vi "Rasnik_Discrepancy.vi"(7 "angle array":string[](array[string]), 8 "pattern":string, 9 "path":path, 10 "Y array":string[](array[string]), 11 "X array":string[](array[string])) -> (1 "angle discrepancy":dbl[](array[numeric]), 2 "Y discrepancy":dbl[](array[numeric]), 3 "X discrepancy":dbl[](array[numeric]))   [LabVIEW 2015]
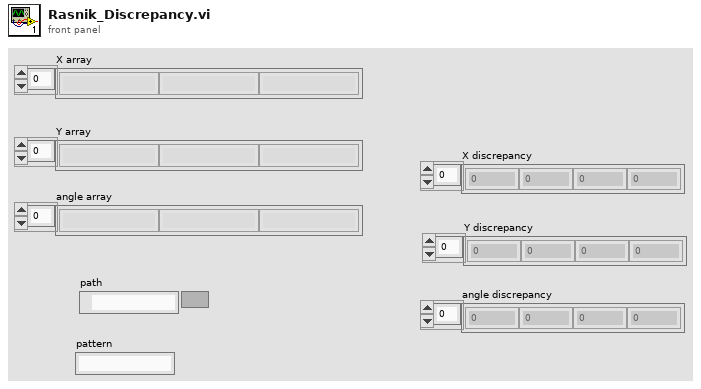
[diagram p1: front panel]
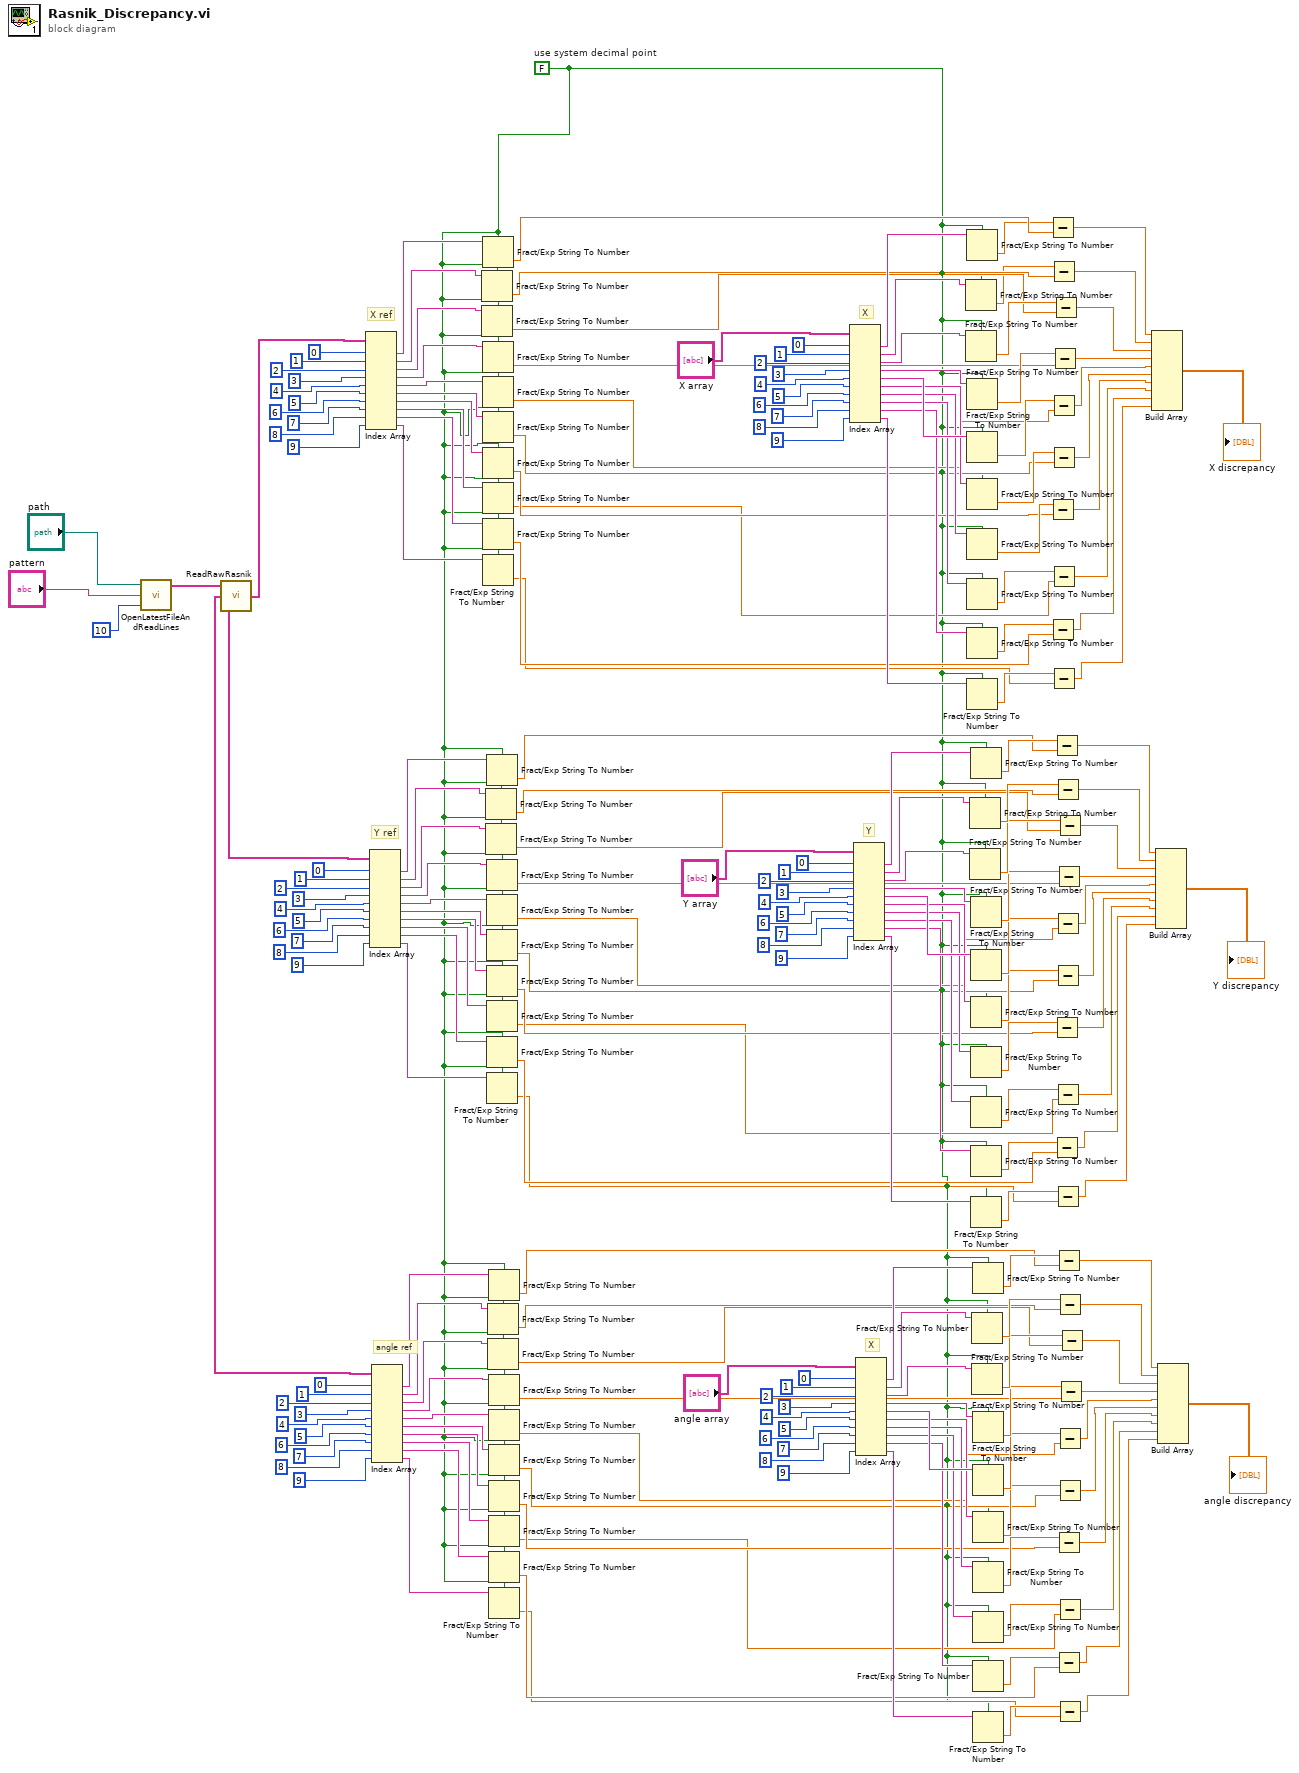
[diagram p0: block diagram]
diagram:
  w1 = FALSE  # use system decimal point
  # "angle ref"
  # "X"
  # "Y ref"
  # "Y"
  # "X ref"
  # "X"
  n1 = call "OpenLatestFileAndReadLines.vi"("No. of lines to read"=10, "pattern"="pattern", "path"="path") -> ("Lines"=w200:string[])  [unwired: 1 in]
  n2 = call "ReadRawRasnik.vi"("Lines"=w200) -> ("X cluster"=w179:string[], "Y cluster"=w77:string[], "angle cluster"=w4:string[])
  n3 = Index Array(array=w179, index #1=0, index #2=1, index #3=2, index #4=3, index #5=4, index #6=5, index #7=6, index #8=7, index #9=8, index #10=9) -> (element #1=w189:string, element #2=w188:string, element #3=w187:string, element #4=w186:string, element #5=w185:string, element #6=w184:string, element #7=w183:string, element #8=w182:string, element #9=w181:string, element #10=w180:string)
  n4 = Index Array(array=w77, index #1=0, index #2=1, index #3=2, index #4=3, index #5=4, index #6=5, index #7=6, index #8=7, index #9=8, index #10=9) -> (element #1=w118:string, element #2=w117:string, element #3=w116:string, element #4=w115:string, element #5=w114:string, element #6=w113:string, element #7=w112:string, element #8=w111:string, element #9=w110:string, element #10=w109:string)
  n5 = Index Array(array=w4, index #1=0, index #2=1, index #3=2, index #4=3, index #5=4, index #6=5, index #7=6, index #8=7, index #9=8, index #10=9) -> (element #1=w45:string, element #2=w44:string, element #3=w43:string, element #4=w42:string, element #5=w41:string, element #6=w40:string, element #7=w39:string, element #8=w38:string, element #9=w37:string, element #10=w36:string)
  n6 = Fract/Exp String To Number(use system decimal point (T)=w1, string=w188) -> (number=w170:dbl)  [unwired: 2 in, 1 out]
  n7 = Fract/Exp String To Number(use system decimal point (T)=w1, string=w187) -> (number=w154:dbl)  [unwired: 2 in, 1 out]
  n8 = Fract/Exp String To Number(use system decimal point (T)=w1, string=w189) -> (number=w150:dbl)  [unwired: 2 in, 1 out]
  n9 = Fract/Exp String To Number(use system decimal point (T)=w1, string=w186) -> (number=w153:dbl)  [unwired: 2 in, 1 out]
  n10 = Fract/Exp String To Number(use system decimal point (T)=w1, string=w185) -> (number=w152:dbl)  [unwired: 2 in, 1 out]
  n11 = Fract/Exp String To Number(use system decimal point (T)=w1, string=w184) -> (number=w151:dbl)  [unwired: 2 in, 1 out]
  n12 = Fract/Exp String To Number(use system decimal point (T)=w1, string=w183) -> (number=w169:dbl)  [unwired: 2 in, 1 out]
  n13 = Fract/Exp String To Number(use system decimal point (T)=w1, string=w182) -> (number=w168:dbl)  [unwired: 2 in, 1 out]
  n14 = Fract/Exp String To Number(use system decimal point (T)=w1, string=w181) -> (number=w167:dbl)  [unwired: 2 in, 1 out]
  n15 = Fract/Exp String To Number(use system decimal point (T)=w1, string=w180) -> (number=w166:dbl)  [unwired: 2 in, 1 out]
  n16 = Fract/Exp String To Number(use system decimal point (T)=w1, string=w117) -> (number=w98:dbl)  [unwired: 2 in, 1 out]
  n17 = Fract/Exp String To Number(use system decimal point (T)=w1, string=w116) -> (number=w82:dbl)  [unwired: 2 in, 1 out]
  n18 = Fract/Exp String To Number(use system decimal point (T)=w1, string=w118) -> (number=w78:dbl)  [unwired: 2 in, 1 out]
  n19 = Fract/Exp String To Number(use system decimal point (T)=w1, string=w115) -> (number=w81:dbl)  [unwired: 2 in, 1 out]
  n20 = Fract/Exp String To Number(use system decimal point (T)=w1, string=w114) -> (number=w80:dbl)  [unwired: 2 in, 1 out]
  n21 = Fract/Exp String To Number(use system decimal point (T)=w1, string=w113) -> (number=w79:dbl)  [unwired: 2 in, 1 out]
  n22 = Fract/Exp String To Number(use system decimal point (T)=w1, string=w112) -> (number=w97:dbl)  [unwired: 2 in, 1 out]
  n23 = Fract/Exp String To Number(use system decimal point (T)=w1, string=w111) -> (number=w96:dbl)  [unwired: 2 in, 1 out]
  n24 = Fract/Exp String To Number(use system decimal point (T)=w1, string=w110) -> (number=w95:dbl)  [unwired: 2 in, 1 out]
  n25 = Fract/Exp String To Number(use system decimal point (T)=w1, string=w109) -> (number=w94:dbl)  [unwired: 2 in, 1 out]
  n26 = Fract/Exp String To Number(use system decimal point (T)=w1, string=w44) -> (number=w25:dbl)  [unwired: 2 in, 1 out]
  n27 = Fract/Exp String To Number(use system decimal point (T)=w1, string=w43) -> (number=w9:dbl)  [unwired: 2 in, 1 out]
  n28 = Fract/Exp String To Number(use system decimal point (T)=w1, string=w45) -> (number=w5:dbl)  [unwired: 2 in, 1 out]
  n29 = Fract/Exp String To Number(use system decimal point (T)=w1, string=w42) -> (number=w8:dbl)  [unwired: 2 in, 1 out]
  n30 = Fract/Exp String To Number(use system decimal point (T)=w1, string=w41) -> (number=w7:dbl)  [unwired: 2 in, 1 out]
  n31 = Fract/Exp String To Number(use system decimal point (T)=w1, string=w40) -> (number=w6:dbl)  [unwired: 2 in, 1 out]
  n32 = Fract/Exp String To Number(use system decimal point (T)=w1, string=w39) -> (number=w24:dbl)  [unwired: 2 in, 1 out]
  n33 = Fract/Exp String To Number(use system decimal point (T)=w1, string=w38) -> (number=w23:dbl)  [unwired: 2 in, 1 out]
  n34 = Fract/Exp String To Number(use system decimal point (T)=w1, string=w37) -> (number=w22:dbl)  [unwired: 2 in, 1 out]
  n35 = Fract/Exp String To Number(use system decimal point (T)=w1, string=w36) -> (number=w21:dbl)  [unwired: 2 in, 1 out]
  n36 = Index Array(array="X array", index #1=0, index #2=1, index #3=2, index #4=3, index #5=4, index #6=5, index #7=6, index #8=7, index #9=8, index #10=9) -> (element #1=w213:string, element #2=w212:string, element #3=w211:string, element #4=w210:string, element #5=w209:string, element #6=w208:string, element #7=w207:string, element #8=w206:string, element #9=w205:string, element #10=w204:string)
  n37 = Index Array(array="Y array", index #1=0, index #2=1, index #3=2, index #4=3, index #5=4, index #6=5, index #7=6, index #8=7, index #9=8, index #10=9) -> (element #1=w138:string, element #2=w137:string, element #3=w136:string, element #4=w135:string, element #5=w134:string, element #6=w133:string, element #7=w132:string, element #8=w131:string, element #9=w130:string, element #10=w129:string)
  n38 = Index Array(array="angle array", index #1=0, index #2=1, index #3=2, index #4=3, index #5=4, index #6=5, index #7=6, index #8=7, index #9=8, index #10=9) -> (element #1=w65:string, element #2=w64:string, element #3=w63:string, element #4=w62:string, element #5=w61:string, element #6=w60:string, element #7=w59:string, element #8=w58:string, element #9=w57:string, element #10=w56:string)
  n39 = Fract/Exp String To Number(use system decimal point (T)=w1, string=w212) -> (number=w2:dbl)  [unwired: 2 in, 1 out]
  n40 = Fract/Exp String To Number(use system decimal point (T)=w1, string=w211) -> (number=w178:dbl)  [unwired: 2 in, 1 out]
  n41 = Fract/Exp String To Number(use system decimal point (T)=w1, string=w213) -> (number=w3:dbl)  [unwired: 2 in, 1 out]
  n42 = Fract/Exp String To Number(use system decimal point (T)=w1, string=w210) -> (number=w177:dbl)  [unwired: 2 in, 1 out]
  n43 = Fract/Exp String To Number(use system decimal point (T)=w1, string=w209) -> (number=w176:dbl)  [unwired: 2 in, 1 out]
  n44 = Fract/Exp String To Number(use system decimal point (T)=w1, string=w208) -> (number=w175:dbl)  [unwired: 2 in, 1 out]
  n45 = Fract/Exp String To Number(use system decimal point (T)=w1, string=w207) -> (number=w174:dbl)  [unwired: 2 in, 1 out]
  n46 = Fract/Exp String To Number(use system decimal point (T)=w1, string=w206) -> (number=w173:dbl)  [unwired: 2 in, 1 out]
  n47 = Fract/Exp String To Number(use system decimal point (T)=w1, string=w205) -> (number=w172:dbl)  [unwired: 2 in, 1 out]
  n48 = Fract/Exp String To Number(use system decimal point (T)=w1, string=w204) -> (number=w171:dbl)  [unwired: 2 in, 1 out]
  n49 = Fract/Exp String To Number(use system decimal point (T)=w1, string=w137) -> (number=w107:dbl)  [unwired: 2 in, 1 out]
  n50 = Fract/Exp String To Number(use system decimal point (T)=w1, string=w136) -> (number=w106:dbl)  [unwired: 2 in, 1 out]
  n51 = Fract/Exp String To Number(use system decimal point (T)=w1, string=w138) -> (number=w108:dbl)  [unwired: 2 in, 1 out]
  n52 = Fract/Exp String To Number(use system decimal point (T)=w1, string=w135) -> (number=w105:dbl)  [unwired: 2 in, 1 out]
  n53 = Fract/Exp String To Number(use system decimal point (T)=w1, string=w134) -> (number=w104:dbl)  [unwired: 2 in, 1 out]
  n54 = Fract/Exp String To Number(use system decimal point (T)=w1, string=w133) -> (number=w103:dbl)  [unwired: 2 in, 1 out]
  n55 = Fract/Exp String To Number(use system decimal point (T)=w1, string=w132) -> (number=w102:dbl)  [unwired: 2 in, 1 out]
  n56 = Fract/Exp String To Number(use system decimal point (T)=w1, string=w131) -> (number=w101:dbl)  [unwired: 2 in, 1 out]
  n57 = Fract/Exp String To Number(use system decimal point (T)=w1, string=w130) -> (number=w100:dbl)  [unwired: 2 in, 1 out]
  n58 = Fract/Exp String To Number(use system decimal point (T)=w1, string=w129) -> (number=w99:dbl)  [unwired: 2 in, 1 out]
  n59 = Fract/Exp String To Number(use system decimal point (T)=w1, string=w64) -> (number=w34:dbl)  [unwired: 2 in, 1 out]
  n60 = Fract/Exp String To Number(use system decimal point (T)=w1, string=w63) -> (number=w33:dbl)  [unwired: 2 in, 1 out]
  n61 = Fract/Exp String To Number(use system decimal point (T)=w1, string=w65) -> (number=w35:dbl)  [unwired: 2 in, 1 out]
  n62 = Fract/Exp String To Number(use system decimal point (T)=w1, string=w62) -> (number=w32:dbl)  [unwired: 2 in, 1 out]
  n63 = Fract/Exp String To Number(use system decimal point (T)=w1, string=w61) -> (number=w31:dbl)  [unwired: 2 in, 1 out]
  n64 = Fract/Exp String To Number(use system decimal point (T)=w1, string=w60) -> (number=w30:dbl)  [unwired: 2 in, 1 out]
  n65 = Fract/Exp String To Number(use system decimal point (T)=w1, string=w59) -> (number=w29:dbl)  [unwired: 2 in, 1 out]
  n66 = Fract/Exp String To Number(use system decimal point (T)=w1, string=w58) -> (number=w28:dbl)  [unwired: 2 in, 1 out]
  n67 = Fract/Exp String To Number(use system decimal point (T)=w1, string=w57) -> (number=w27:dbl)  [unwired: 2 in, 1 out]
  n68 = Fract/Exp String To Number(use system decimal point (T)=w1, string=w56) -> (number=w26:dbl)  [unwired: 2 in, 1 out]
  n69 = Subtract(x=w3, y=w150) -> (x-y=w165:dbl)
  n70 = Subtract(x=w174, y=w169) -> (x-y=w159:dbl)
  n71 = Subtract(x=w172, y=w167) -> (x-y=w157:dbl)
  n72 = Subtract(x=w2, y=w170) -> (x-y=w164:dbl)
  n73 = Subtract(x=w176, y=w152) -> (x-y=w161:dbl)
  n74 = Subtract(x=w175, y=w151) -> (x-y=w160:dbl)
  n75 = Subtract(x=w173, y=w168) -> (x-y=w158:dbl)
  n76 = Subtract(x=w171, y=w166) -> (x-y=w156:dbl)
  n77 = Subtract(x=w177, y=w153) -> (x-y=w162:dbl)
  n78 = Subtract(x=w178, y=w154) -> (x-y=w163:dbl)
  n79 = Subtract(x=w108, y=w78) -> (x-y=w93:dbl)
  n80 = Subtract(x=w102, y=w97) -> (x-y=w87:dbl)
  n81 = Subtract(x=w100, y=w95) -> (x-y=w85:dbl)
  n82 = Subtract(x=w107, y=w98) -> (x-y=w92:dbl)
  n83 = Subtract(x=w104, y=w80) -> (x-y=w89:dbl)
  n84 = Subtract(x=w103, y=w79) -> (x-y=w88:dbl)
  n85 = Subtract(x=w101, y=w96) -> (x-y=w86:dbl)
  n86 = Subtract(x=w99, y=w94) -> (x-y=w84:dbl)
  n87 = Subtract(x=w105, y=w81) -> (x-y=w90:dbl)
  n88 = Subtract(x=w35, y=w5) -> (x-y=w20:dbl)
  n89 = Subtract(x=w29, y=w24) -> (x-y=w14:dbl)
  n90 = Subtract(x=w27, y=w22) -> (x-y=w12:dbl)
  n91 = Subtract(x=w106, y=w82) -> (x-y=w91:dbl)
  n92 = Subtract(x=w34, y=w25) -> (x-y=w19:dbl)
  n93 = Subtract(x=w31, y=w7) -> (x-y=w16:dbl)
  n94 = Subtract(x=w30, y=w6) -> (x-y=w15:dbl)
  n95 = Subtract(x=w28, y=w23) -> (x-y=w13:dbl)
  n96 = Subtract(x=w26, y=w21) -> (x-y=w11:dbl)
  n97 = Subtract(x=w32, y=w8) -> (x-y=w17:dbl)
  n98 = Subtract(x=w33, y=w9) -> (x-y=w18:dbl)
  n99 = Build Array(w165, w164, w163, w162, w161, w160, w159, w158, w157, w156) -> (→"X discrepancy":dbl[])
  n100 = Build Array(w93, w92, w91, w90, w89, w88, w87, w86, w85, w84) -> (→"Y discrepancy":dbl[])
  n101 = Build Array(w20, w19, w18, w17, w16, w15, w14, w13, w12, w11) -> (→"angle discrepancy":dbl[])
